vi "DataAcqStatus.vi"(0 "ABORT":bool) -> ()   [LabVIEW 2022 SP3]
uses:
  ScanningControl/Digitizers/GaGe/-GageUtils/GageGlobals.vi
panel:
  out "Shot Number":i32
  out "Percenrt Complete":dbl(slide) scale=0.0..100.0
  out "# Firings":u16=1 min=1
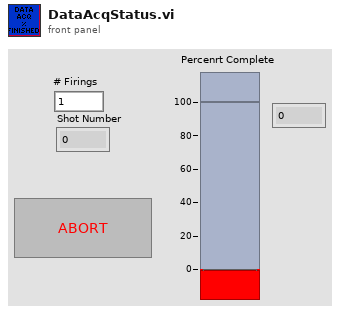
[diagram p1: front panel]
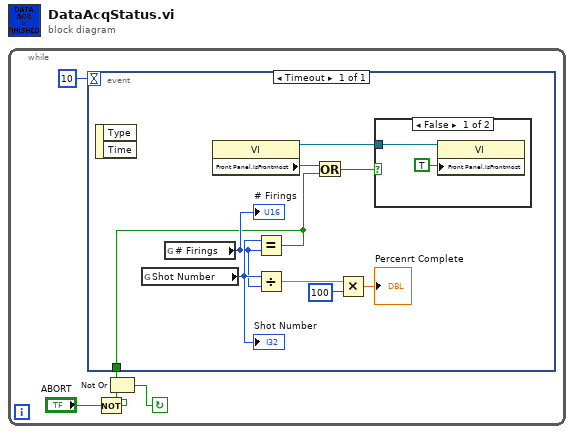
[diagram p0: block diagram]
diagram:
  n1 = while {
    stop <- w2 continue-if-true
    n2 = event shown="[0] Timeout" {
      selector: _ -> [_]
      dyn-events: _ -> [_]
      timeout: 10 -> [_]
      tunnel: [w6] -> w1
      event Timeout {
        n3 = event-data() -> ()  [unwired: 1 in, 2 out]
        n4 = global read "GageGlobals.vi" "Shot Number"() -> (w10:i32)
        "Shot Number" <- w10
        n5 = global read "GageGlobals.vi" "# Firings"() -> (w9:u16)
        "# Firings" <- w9
        n6 = property class="VI"() -> (reference out=w11:refnum<vi>, "Front Panel.IsFrontmost"=w8:bool)  [unwired: 2 in, 1 out]
        n7 = Equal?(x=w10, y=w9) -> (x = y?=w6:bool)
        n8 = Divide(x=w10, y=w9) -> (x/y=w14:dbl)
        n9 = Or(x=w8, y=w6) -> (x .or. y?=w7:bool)
        n10 = Multiply(x=w14, y=100) -> (x*y=→"Percenrt Complete":dbl)
        n11 = case shown="False" w7 {
          tunnel: w11 -> [w16 _]
          frame False {
            n12 = property class="VI"(reference=w16, "Front Panel.IsFrontmost"=TRUE) -> ()  [unwired: 1 in, 2 out]
          }
          frame True {
          }
        }
      }
    }
    n13 = Not(x="ABORT") -> (.not. x?=w3:bool)
    n14 = Not Or(1:w3, 2:w1) -> (0:w2:bool)
  }
